vi "LabVIEW-ini Config.vi"(7 "Global Config":T1, 8 "error in":errorcluster, 10 "ini Name (LabVIEW.ini)":path=path "LabVIEW.ini", 11 "LabVIEW Install Folder":path=path "C:/Program Files (x86)/National Instruments/LabVIEW 2021") -> (0 "error out":errorcluster)   [LabVIEW 2021]
uses:
  Global Config.ctl
  ini Entry.ctl
  VIPM.ctl
  <vilib>/Utility/error.llb/Error Cluster From Error Code.vi
  <vilib>/Utility/config.llb/Write Key (Boolean).vi
  <vilib>/Utility/config.llb/Write Key (String).vi
  <vilib>/Utility/config.llb/Write Key (Path).vi
  <vilib>/Utility/config.llb/Write Key (I32).vi
  <vilib>/Utility/config.llb/Write Key (U32).vi
  <vilib>/Utility/config.llb/Write Key (Double).vi
  <vilib>/ErrorRing/Error Ring.xnode
  <vilib>/Utility/config.llb/NI_LVConfig.lvlib
  <vilib>/Utility/Data Type/NI_Data Type.lvlib
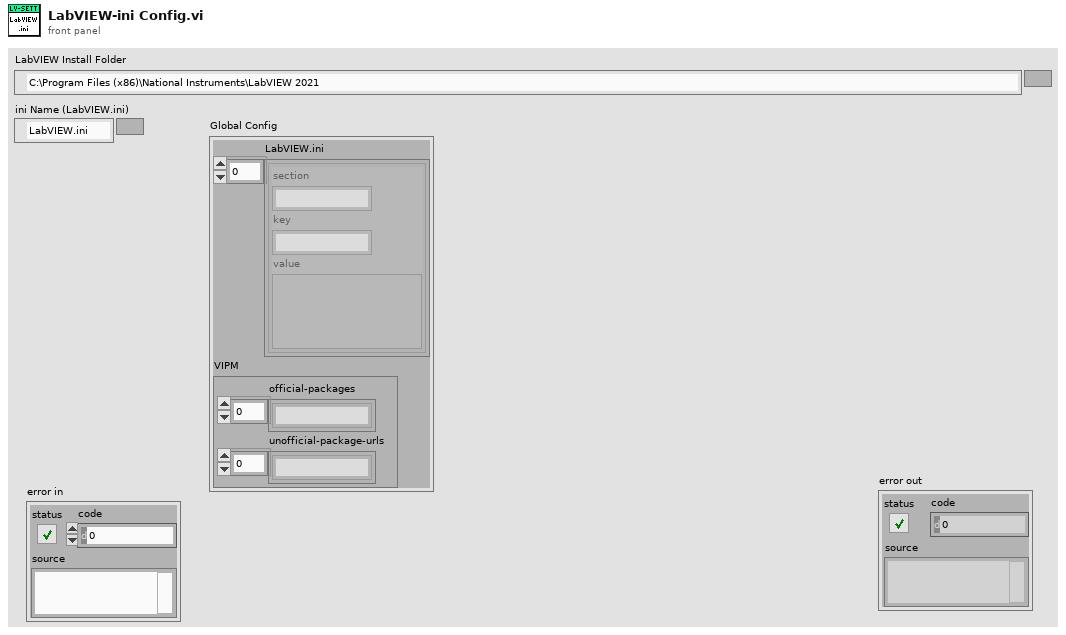
[diagram p1: front panel]
types:
  T1 = typedef "Global Config.ctl" = cluster{"LabVIEW.ini":T2[], "VIPM":T3}
  T2 = typedef "ini Entry.ctl" = cluster{"section":string, "key":string, "value":variant}
  T3 = typedef "VIPM.ctl" = cluster{"official-packages":string[], "unofficial-package-urls":string[]}
  T4 = typedef "NI_LVConfig.lvlib/Config Data RefNum.ctl" = refnum<k1>
  T5 = typedef "NI_Data Type.lvlib/Data Type.ctl" = enum8{"Invalid Type", "Void", "I8", "I16", "I32", "I64", "U8", "U16", "U32", "U64", "Single Float", "Double Float", "Extended Float", "Single Complex", "Double Complex", "Extended Complex", "Enum U8", "Enum U16", "Enum U32", "Enum U64", "Single Float With Unit", "Double Float With Unit", "Extended Float With Unit", "Single Complex with Unit", "Double Complex with Unit", "Extended Complex with Unit", "Boolean", "String", "Path", "Picture", "Tag", "Array", "Cluster", "Variant", "LV Variant", "Waveform", "Timestamp", "Digital Waveform", "Digital Data", "ExpressData", "Refnum", "External Data", "VI", "Poly VI", "LabVIEW Class Instance", "Fixed Point", "Set Collection", "Map Collection"}
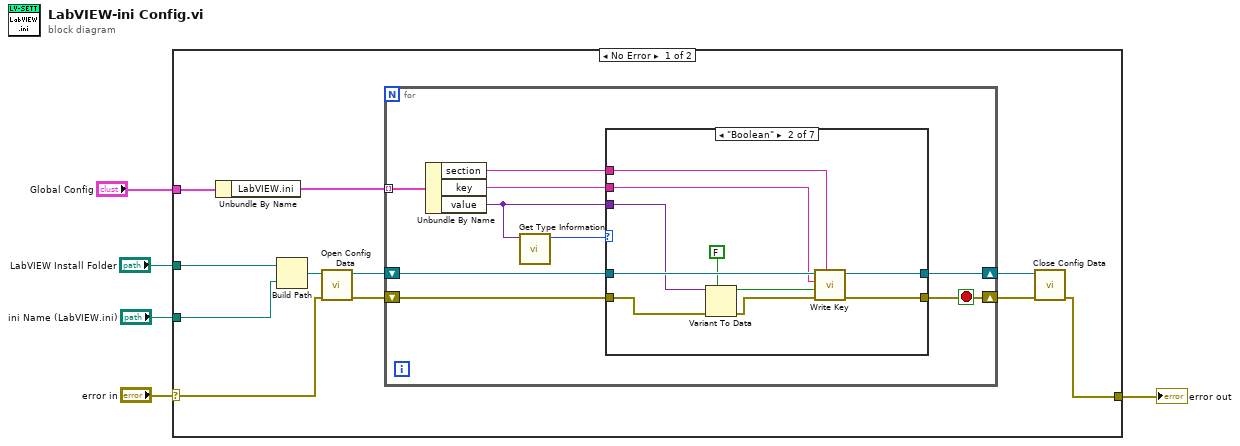
[diagram p0: block diagram]
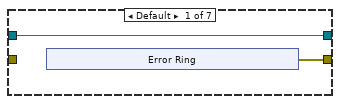
[diagram p2: hidden frame]
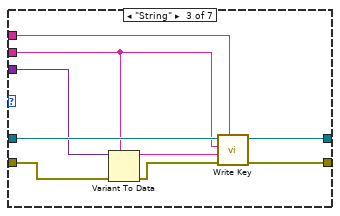
[diagram p3: hidden frame]
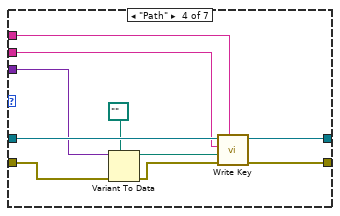
[diagram p4: hidden frame]
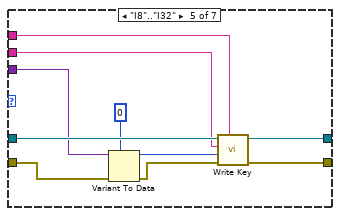
[diagram p5: hidden frame]
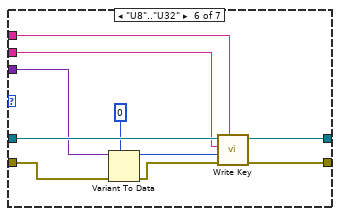
[diagram p6: hidden frame]
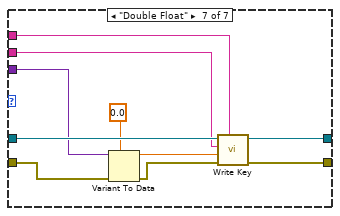
[diagram p7: hidden frame]
diagram:
  n1 = case shown="No Error" "error in" {
    selector: "error in" -> [w10 w91]
    tunnel: [w9 w91] -> w4
    tunnel: "LabVIEW Install Folder" -> [w16 _]
    tunnel: "Global Config" -> [w8 _]
    tunnel: "ini Name (LabVIEW.ini)" -> [w6 _]
    frame No Error {
      n2 = Unbundle By Name(w8) -> ("LabVIEW.ini"=w7:T2[])
      n3 = Build Path(base path=w16, name or relative path=w6) -> (appended path=w15:path)
      n4 = call <vilib>:"Open Config Data.vi"("error in (no error)"=w10, "configuration file path"=w15) -> ("error out"=w13:errorcluster, "refnum"=w14:T4)  [unwired: 7 in, 1 out]
      n5 = for {
        shift-right: [w23] -> w12
        shift-left: w14 -> [w24]
        shift-right: [w17] -> w11
        shift-left: w13 -> [w25]
        tunnel: w7 -> [w22] mode=indexing
        stop <- w17 stop-if-true
        n6 = Unbundle By Name(w22) -> ("section"=w21:string, "key"=w20:string, "value"=w19:variant)
        n7 = call <vilib>:"Get Type Information.vi"("variant"=w19) -> ("type"=w18:T5)  [unwired: 6 in, 4 out]
        n8 = case shown="\"Boolean\"" w18 {
          tunnel: w25 -> [_ w34 w44 w54 w64 w74 w84]
          tunnel: [w27 w41 w50 w60 w70 w80 w90] -> w17
          tunnel: w24 -> [w26 w40 w49 w59 w69 w79 w89]
          tunnel: [w26 w39 w48 w58 w68 w78 w88] -> w23
          tunnel: w21 -> [_ w38 w47 w57 w67 w77 w87]
          tunnel: w20 -> [_ w37 w42 w52 w62 w72 w82]
          tunnel: w19 -> [_ w33 w43 w53 w63 w73 w83]
          frame Default {
            n9 = xnode "Error Ring"() -> ("error out"=w27:errorcluster)
          }
          frame "Boolean" {
            n10 = Variant To Data(error in=w34, type=FALSE, Variant=w33) -> (data=w36:bool, error out=w35:errorcluster)
            n11 = call-poly <vilib>:"Write Key.vi"("section"=w38, "error in (no error)"=w35, "value"=w36, "key"=w37, "refnum"=w40) -> ("error out"=w41:errorcluster, "refnum out"=w39:T4)  [unwired: 4 in, 1 out]
          }
          frame "String" {
            n12 = Variant To Data(error in=w44, type=w42, Variant=w43) -> (data=w46:string, error out=w45:errorcluster)
            n13 = call-poly <vilib>:"Write Key.vi"("section"=w47, "error in (no error)"=w45, "value"=w46, "key"=w42, "refnum"=w49) -> ("error out"=w50:errorcluster, "refnum out"=w48:T4)  [unwired: 4 in, 1 out]
          }
          frame "Path" {
            n14 = Variant To Data(error in=w54, type=path "", Variant=w53) -> (data=w56:path, error out=w55:errorcluster)
            n15 = call-poly <vilib>:"Write Key.vi"("section"=w57, "error in (no error)"=w55, "value"=w56, "key"=w52, "refnum"=w59) -> ("error out"=w60:errorcluster, "refnum out"=w58:T4)  [unwired: 4 in, 1 out]
          }
          frame "I8".."I32" {
            n16 = Variant To Data(error in=w64, type=0, Variant=w63) -> (data=w66:i32, error out=w65:errorcluster)
            n17 = call-poly <vilib>:"Write Key.vi"("section"=w67, "error in (no error)"=w65, "value"=w66, "key"=w62, "refnum"=w69) -> ("error out"=w70:errorcluster, "refnum out"=w68:T4)  [unwired: 4 in, 1 out]
          }
          frame "U8".."U32" {
            n18 = Variant To Data(error in=w74, type=u32 0, Variant=w73) -> (data=w76:u32, error out=w75:errorcluster)
            n19 = call-poly <vilib>:"Write Key.vi"("section"=w77, "error in (no error)"=w75, "value"=w76, "key"=w72, "refnum"=w79) -> ("error out"=w80:errorcluster, "refnum out"=w78:T4)  [unwired: 4 in, 1 out]
          }
          frame "Double Float" {
            n20 = Variant To Data(error in=w84, type=0.0, Variant=w83) -> (data=w86:dbl, error out=w85:errorcluster)
            n21 = call-poly <vilib>:"Write Key.vi"("section"=w87, "error in (no error)"=w85, "value"=w86, "key"=w82, "refnum"=w89) -> ("error out"=w90:errorcluster, "refnum out"=w88:T4)  [unwired: 4 in, 1 out]
          }
        }
      }
      n22 = call <vilib>:"Close Config Data.vi"("error in (no error)"=w11, "refnum"=w12) -> ("error out"=w9:errorcluster)  [unwired: 8 in, 1 out]
    }
    frame Error {
    }
  }
  "error out" <- w4
